vi "InitializeIntensityGraph.vi"(10 "Intensity Graph 1 in":refnum<vi>, 11 "IntensityGraph 2 in":refnum<vi>) -> ()   [LabVIEW 2022 SP3]
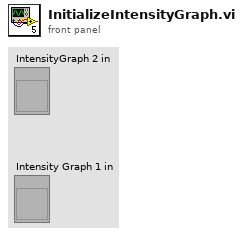
[diagram p1: front panel]
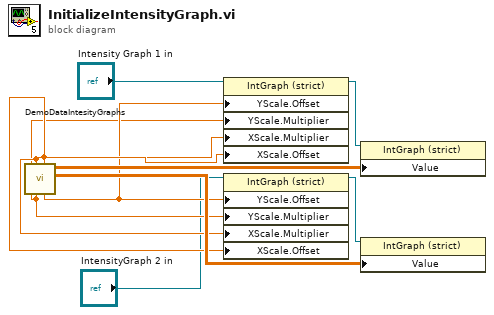
[diagram p0: block diagram]
diagram:
  n1 = call "DemoDataIntesityGraphs.vi"() -> ("Array 2"=w10:dbl[][], "Array"=w8:dbl[][], "y offset"=w5:dbl, "x offset"=w6:dbl, "Y multi"=w3:dbl, "x multi"=w4:dbl)  [unwired: 6 in]
  n2 = property class="IntGraph (strict)"(reference="Intensity Graph 1 in", "YScale.Offset"=w5, "YScale.Multiplier"=w3, "XScale.Multiplier"=w4, "XScale.Offset"=w6) -> (reference out=w7:refnum<vi>)  [unwired: 1 in, 1 out]
  n3 = property class="IntGraph (strict)"(reference="IntensityGraph 2 in", "YScale.Offset"=w5, "YScale.Multiplier"=w3, "XScale.Multiplier"=w4, "XScale.Offset"=w6) -> (reference out=w9:refnum<vi>)  [unwired: 1 in, 1 out]
  n4 = property class="IntGraph (strict)"(reference=w7, "Value"=w8) -> ()  [unwired: 1 in, 2 out]
  n5 = property class="IntGraph (strict)"(reference=w9, "Value"=w10) -> ()  [unwired: 1 in, 2 out]
